vi "DCP551.vi"() -> ()   [LabVIEW 2010]
uses:
  Segment 1 to 99.ctl
  DCP551.lvlib
panel:
  in  "Segment 0":T1={"Start"=enum."Non PV start", "Cycle data"=0, "Pattern link data"=0, "Tag data"="12345678"}
  in  "Segment 1 to 99":T2[](array[typedef])
  in  "Tag data":string="12345678"
  in  "Pattern link data":i32
  in  "Cycle data":i32
  in  "Start":T3(ring)
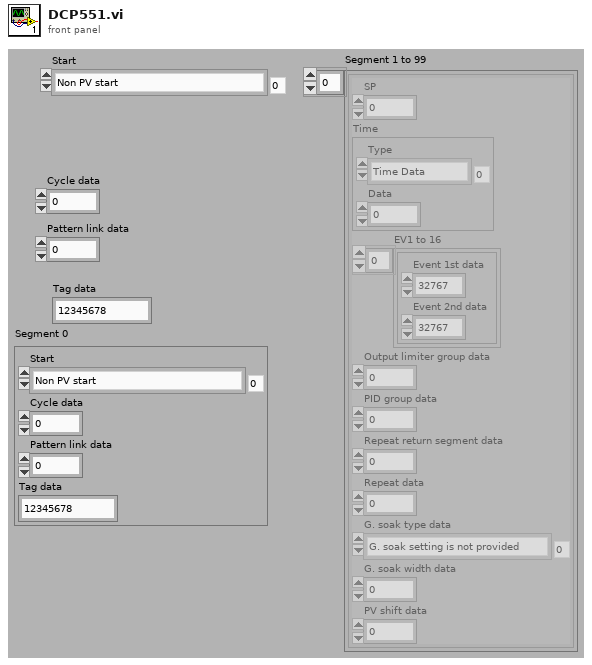
[diagram p1: front panel]
types:
  T1 = cluster{"Start":enum16{"Non PV start", "Upward PV tart", "Downward PV start", "Either upward of downward PV start"}, "Cycle data":i32, "Pattern link data":i32, "Tag data":string}
  T2 = typedef "DCP551.lvlib/Segment.ctl" = cluster{"SP":dbl, "Time":cluster{"Type":enum16{"Time Data", "delta Dtada", "SP Data"}, "Data":i32}, "EV1 to 16":cluster{"Event 1st data":i32, "Event 2nd data":i32}[], "Output limiter group data":i32, "PID group data":i32, "Repeat return segment data":i32, "Repeat data":i32, "G. soak type data":enum16{"G. soak setting is not provided", "Segment start point", "Segment end point", "Total segment"}, "G. soak width data":i32, "PV shift data":i32}
  T3 = enum16{"Non PV start", "Upward PV tart", "Downward PV start", "Either upward of downward PV start"}
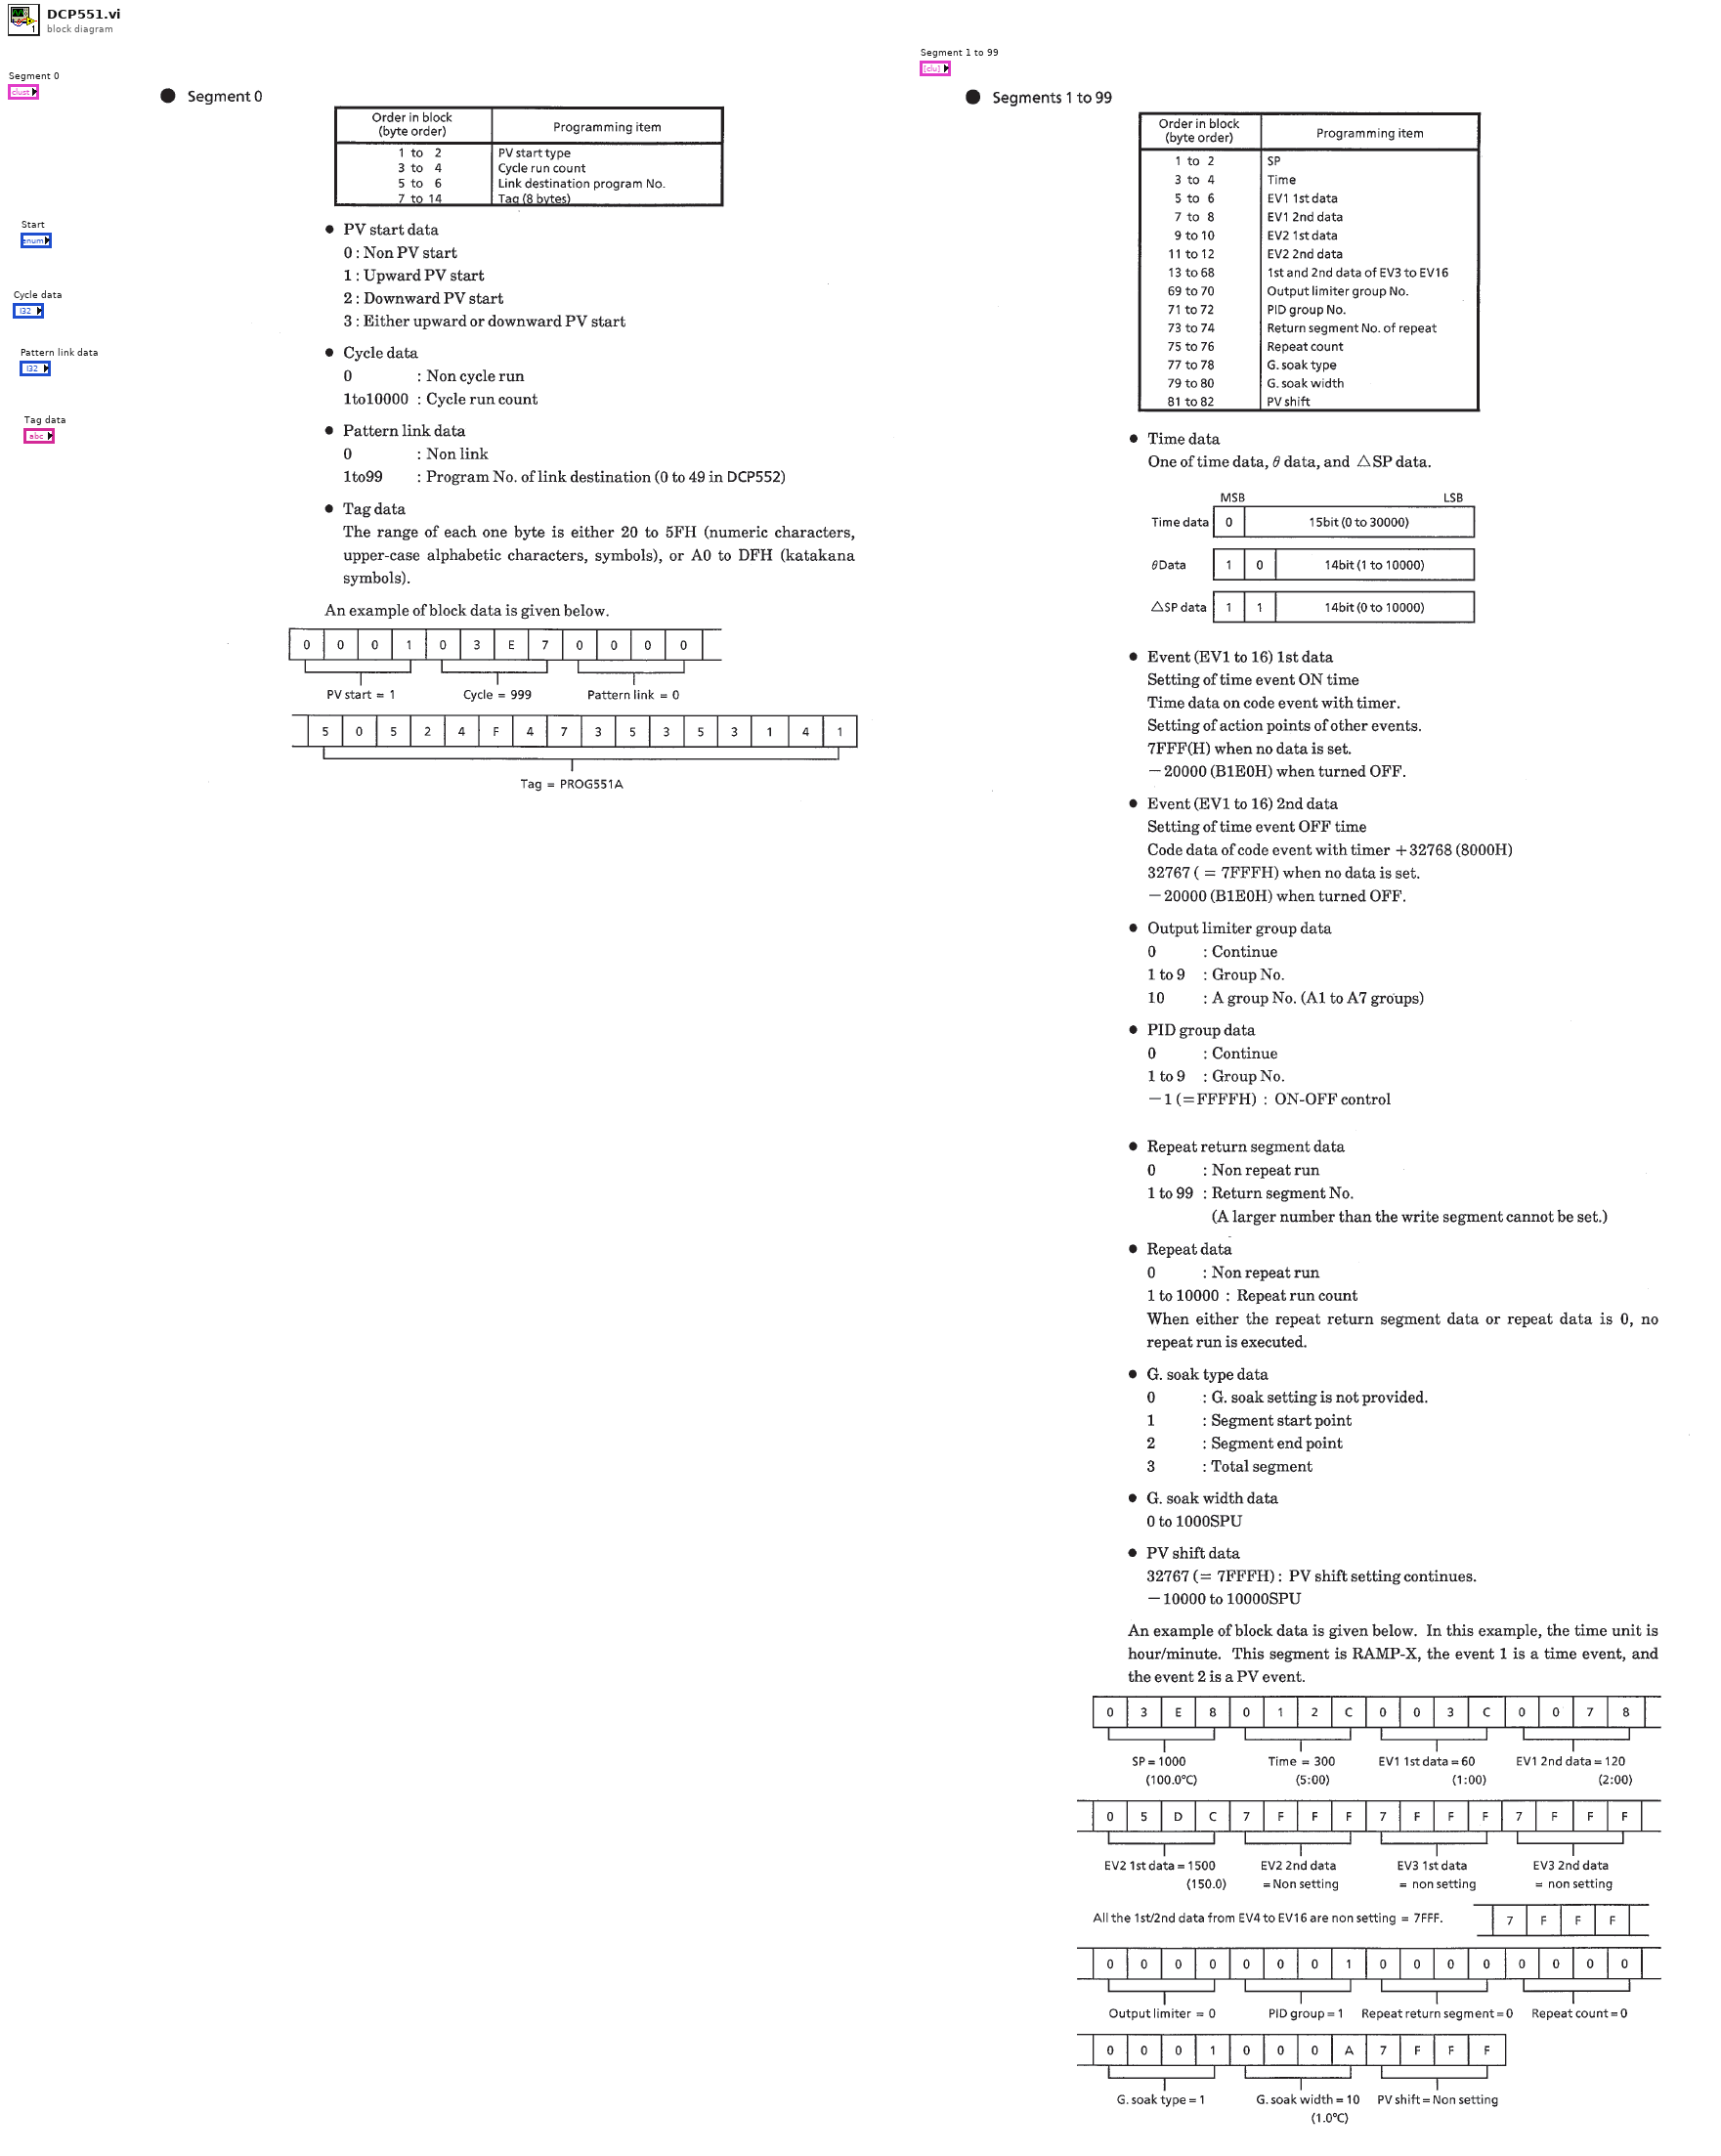
[diagram p0: block diagram]
diagram:
